vi "CSM-RunScript.vi"(7 "LabVIEW Web Service Request":refnum<class "Web Request.lvclass">) -> ()   [LabVIEW 2020]
uses:
  <vilib>/wsapi/Web Request.lvclass
  <userlib>/_NEVSTOP/Communicable State Machine(CSM)/AdvanceAPI/CSM - Convert Error to Argument.vi
  <userlib>/_NEVSTOP/Communicable State Machine(CSM)/_Support/GlobalEvent/GEvt-Generate with Rule Check.vi
  <userlib>/_NEVSTOP/Communicable State Machine(CSM)/_Support/GlobalEvent/Cache-GEvt Refs.vi
  <userlib>/_NEVSTOP/Communicable State Machine(CSM)/AdvanceAPI/CSM - Make String Arguments Safe.vi
  <userlib>/_NEVSTOP/Communicable State Machine(CSM)/_Support/ChangeFlag/FlagInstance-GEvt Refs.vi
  <userlib>/_NEVSTOP/Communicable State Machine(CSM)/AdvanceAPI/CSM - Keywords.vi
  <userlib>/_NEVSTOP/Communicable State Machine(CSM)/_Support/ChangeFlag/ChangeFlag-Read.vi
  <userlib>/_NEVSTOP/Communicable State Machine(CSM)/_Support/ChangeFlag/ChangeFlagDB.vi
  <userlib>/_NEVSTOP/Communicable State Machine(CSM)/_Support/GlobalEvent/FGV-GlobalEventRef(lvlibp).vi
  <userlib>/_NEVSTOP/Communicable State Machine(CSM)/_Support/GlobalEvent/FGV-GlobalEventQueues(lvlibp).vi
  <userlib>/_NEVSTOP/Communicable State Machine(CSM)/_Support/GlobalEvent/GEvt-Valid Subscribers.vi
  <userlib>/_NEVSTOP/Communicable State Machine(CSM)/_Support/GlobalEvent/LogFilter/LogFilter - Check.vi
  <userlib>/_NEVSTOP/Communicable State Machine(CSM)/_Support/GlobalEvent/LogFilter/LogFilter.lvclass
  <userlib>/_NEVSTOP/Communicable State Machine(CSM)/Communicable State Machine.lvlib
  CSM WebService.lvlib
panel:
  # "Use the Web Service Request input terminal to call the VIs on the Web Services palette. Do not remove it from the connector pane unless you don't need access to the palette."
  # "Each additional control wired to the connector pane will be available as an input in the URL. To include an indicator in terminal-mode output (the default setting), it must also be wired to the connector pane."
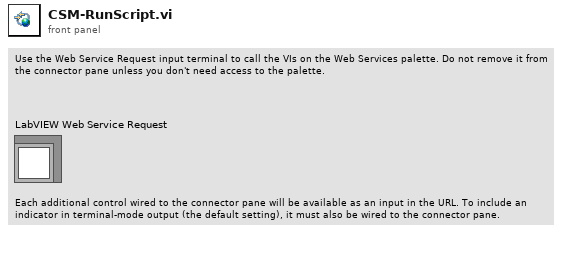
[diagram p1: front panel]
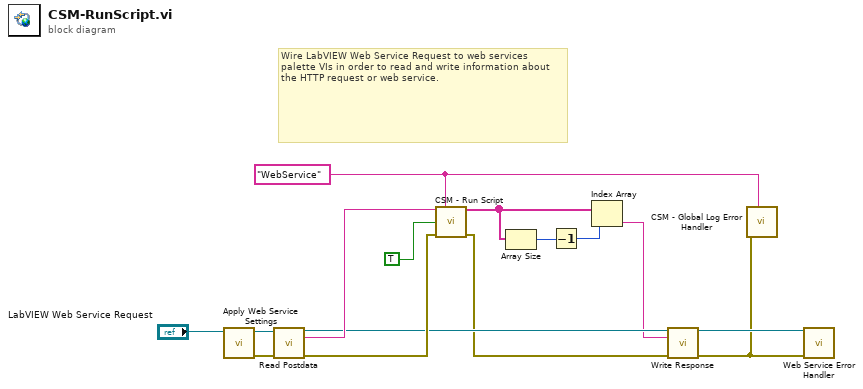
[diagram p0: block diagram]
diagram:
  w9 = "WebService" ("Current Module(\"\" to generate a ID)")
  # "Wire LabVIEW Web Service Request to web services palette VIs in order to read and write information about the HTTP request or web service."
  n1 = call "Apply Web Service Settings.vi"("LabVIEW Web Service Request"="LabVIEW Web Service Request") -> ("error out"=w13:errorcluster, "LabVIEW Web Service Request out"=w14:refnum<class "Web Request.lvclass">)  [unwired: 9 in]
  n2 = call <vilib>:"Read Postdata.vi"("LabVIEW Web Service Request"=w14, "error in (no error)"=w13) -> ("LabVIEW Web Service Request out"=w8:refnum<class "Web Request.lvclass">, "postdata"=w12:string, "error out"=w11:errorcluster)  [unwired: 11 in]
  n3 = call <userlib>:"CSM - Run Script.vi"("CSM Scripts"=w12, "Current Module (\"\" to Generate an ID)"=w9, "Continue If Error? (F)"=TRUE ("Continue If Error?(F)"), "error in (no error)"=w11) -> ("Response"=w1:string[], "error out"=w7:errorcluster)  [unwired: 9 in, 1 out]
  n4 = Array Size(array=w1) -> (size(s)=w2:i32)
  n5 = Decrement(x=w2) -> (x-1=w3:i32)
  n6 = Index Array(array=w1, index=w3) -> (element=w4:string)
  n7 = call <vilib>:"Write Response.vi"("LabVIEW Web Service Request"=w8, "response string"=w4, "error in (no error)"=w7) -> ("LabVIEW Web Service Request out"=w6:refnum<class "Web Request.lvclass">, "error out"=w5:errorcluster)  [unwired: 11 in]
  n8 = call <userlib>:"CSM - Global Log Error Handler.vi"("Place (\"\" to Use VI's Name)"=w9, "Error In"=w5) -> ()  [unwired: 9 in, 1 out]
  n9 = call "Web Service Error Handler.vi"("LabVIEW Web Service Request"=w6, "error in (no error)"=w5) -> ()  [unwired: 12 in, 2 out]
